vi "Baidu_Map_GET_W.vi"() -> ()   [LabVIEW 2013]
uses:
  <vilib>/httpClient/LabVIEWHTTPClient.lvlib
panel:
  out "loops":i32
  in  "stop":bool
  out "error out":errorcluster
  out "hour":dbl
  out "minute":dbl
  out "toll_distance":string
  out "tollfee":string
  out "duration":string
  out "distance":string
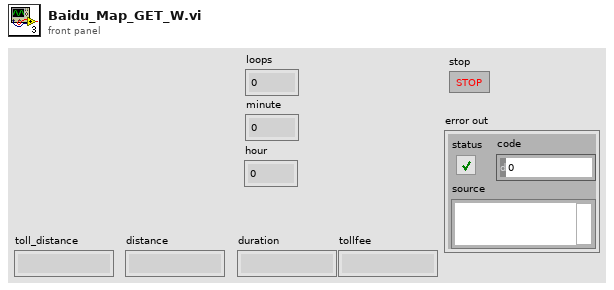
[diagram p1: front panel]
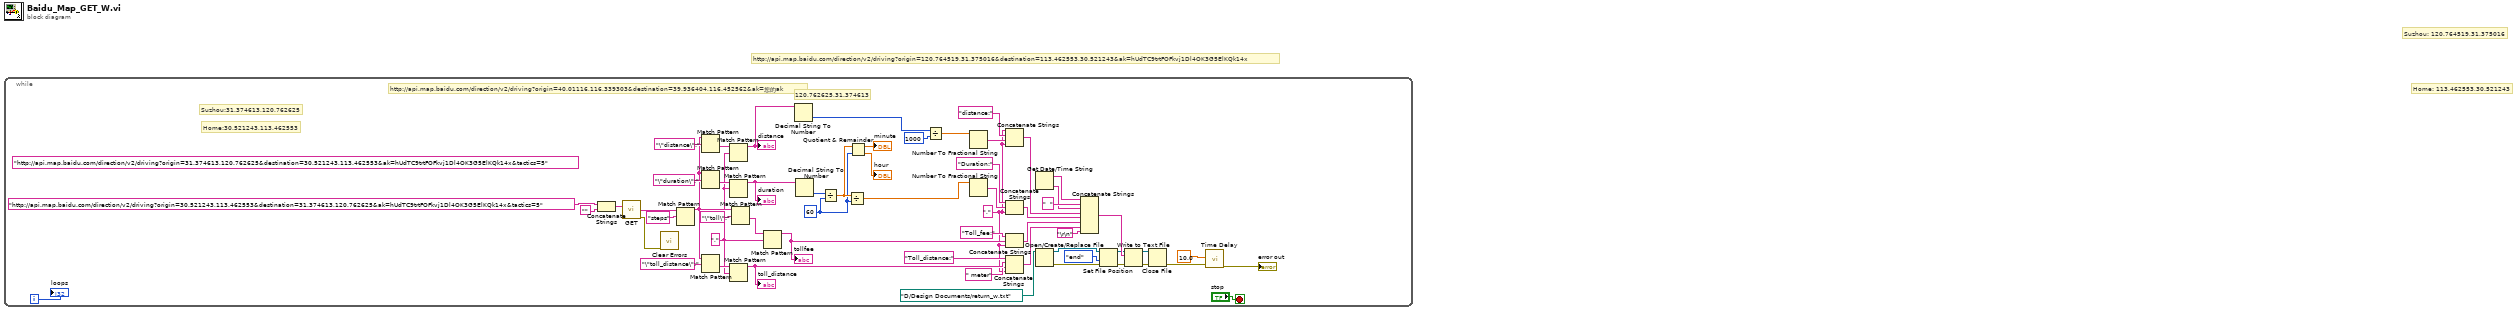
[diagram p0: block diagram]
diagram:
  # "http://api.map.baidu.com/direction/v2/driving?origin=40.01116,116.339303&destination=39.936404,116.452562&ak=您的ak"
  # "Home: 113.462553,30.521243"
  # "Suzhou: 120.764519,31.375016"
  # "http://api.map.baidu.com/direction/v2/driving?origin=120.764519,31.375016&destination=113.462553,30.521243&ak=hUdTC9trtFOFkvj1Dl4OK3G5ElKQk14x"
  n1 = while {
    i -> [w3]
    stop <- "stop" stop-if-true
    (unwired) "http://api.map.baidu.com/direction/v2/driving?origin=31.374613,120.762625&destination=30.521243,113.462553&ak=hUdTC9trtFOFkvj1Dl4OK3G5ElKQk14x&tactics=5" ("string")
    w22 = "," ("regular expression")
    w31 = 60 ("y")
    w47 = "," ("regular expression")
    # "Home:30.521243,113.462553"
    # "Suzhou:31.374613,120.762625"
    # "120.762625,31.374613"
    n2 = Concatenate Strings("http://api.map.baidu.com/direction/v2/driving?origin=30.521243,113.462553&destination=31.374613,120.762625&ak=hUdTC9trtFOFkvj1Dl4OK3G5ElKQk14x&tactics=5" ("string"), "") -> (w59:string)
    n3 = call <vilib>:"GET.vi"("url"=w59) -> ("body"=w8:string, "error out"=w2:errorcluster)  [unwired: 11 in, 2 out]
    n4 = call <vilib>:"Clear Errors.vi"("error in (no error)"=w2) -> ()  [unwired: 6 in, 1 out]
    n5 = Match Pattern(string=w8, regular expression="steps") -> (before substring=w49:string)  [unwired: 1 in, 3 out]
    n6 = Match Pattern(string=w49, regular expression="\"distance\":") -> (after substring=w55:string)  [unwired: 1 in, 3 out]
    n7 = Match Pattern(string=w49, regular expression="\"duration\":") -> (after substring=w53:string)  [unwired: 1 in, 3 out]
    n8 = Match Pattern(string=w49, regular expression="\"toll_distance\":") -> (after substring=w48:string)  [unwired: 1 in, 3 out]
    n9 = Match Pattern(string=w55, regular expression=w47) -> (before substring=w39:string)  [unwired: 1 in, 3 out]
    "distance" <- w39
    n10 = Match Pattern(string=w53, regular expression=w47) -> (before substring=w46:string)  [unwired: 1 in, 3 out]
    "duration" <- w46
    n11 = Match Pattern(string=w48, regular expression=w47) -> (before substring=w24:string)  [unwired: 1 in, 3 out]
    "toll_distance" <- w24
    n12 = Match Pattern(string=w49, regular expression="\"toll\":") -> (after substring=w51:string)  [unwired: 1 in, 3 out]
    n13 = Match Pattern(string=w51, regular expression=w47) -> (before substring=w26:string)  [unwired: 1 in, 3 out]
    "tollfee" <- w26
    n14 = Decimal String To Number(string=w39) -> (number=w38:i32)  [unwired: 2 in, 1 out]
    n15 = Decimal String To Number(string=w46) -> (number=w45:i32)  [unwired: 2 in, 1 out]
    n16 = Divide(x=w45, y=w31) -> (x/y=w32:dbl)
    n17 = Divide(x=w32, y=w31) -> (x/y=w30:dbl)
    n18 = Quotient & Remainder(x=w32, y=w31) -> (x-y*floor(x/y)=→"minute":dbl, floor(x/y)=→"hour":dbl)
    n19 = Divide(x=w38, y=1000) -> (x/y=w36:dbl)
    n20 = Number To Fractional String(number=w36) -> (F-format string=w34:string)  [unwired: 3 in]
    n21 = Number To Fractional String(number=w30) -> (F-format string=w28:string)  [unwired: 3 in]
    n22 = Concatenate Strings(w22, "distance:" ("string"), w34, w22) -> (w33:string)
    n23 = Concatenate Strings("Duration:" ("string"), w28, w22) -> (w21:string)
    n24 = Concatenate Strings("Toll_fee:" ("string"), w26, w22) -> (w20:string)
    n25 = Concatenate Strings("Toll_distance:" ("string"), w24, " meter" ("string"), w22) -> (w19:string)
    n26 = Get Date/Time String() -> (date string=w42:string, time string=w40:string)  [unwired: 3 in]
    n27 = Open/Create/Replace File(file path (use dialog)=path "D:/Design Documents/return_w.txt") -> (refnum out=w15:refnum<file>, error out=w13:errorcluster)  [unwired: 5 in, 1 out]
    n28 = Concatenate Strings(w42, "  " ("string"), w40, w33, w21, w20, w19, "\r\n") -> (w16:string)
    n29 = Set File Position(refnum=w15, from (0:start)=enum16{"start", "end", "current"}."end", error in=w13) -> (refnum out=w14:refnum<file>, error out=w11:errorcluster)  [unwired: 1 in]
    n30 = Write to Text File(file (use dialog)=w14, text=w16, error in=w11) -> (refnum out=w10:refnum<file>, error out=w9:errorcluster)  [unwired: 1 in, 1 out]
    n31 = Close File(refnum=w10, error in=w9) -> (error out=w6:errorcluster)  [unwired: 1 out]
    n32 = call "Time Delay"("error in (no error)"=w6, "Delay Time (s)"=10.0) -> ("error out"=→"error out":errorcluster)  [unwired: 9 in]
    "loops" <- w3
  }
